vi "Terminal_Log_In_Judge.vi"(8 "密码":string, 9 "用户名":string, 10 "用户个数":dbl, 11 "用户名密码信息":string[][](table)) -> (3 "用户名密码匹配":bool)   [LabVIEW 2014]
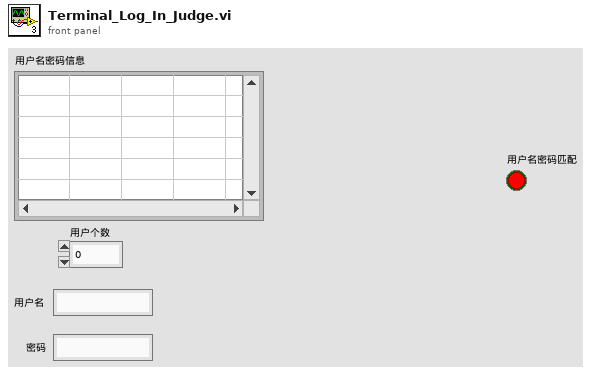
[diagram p1: front panel]
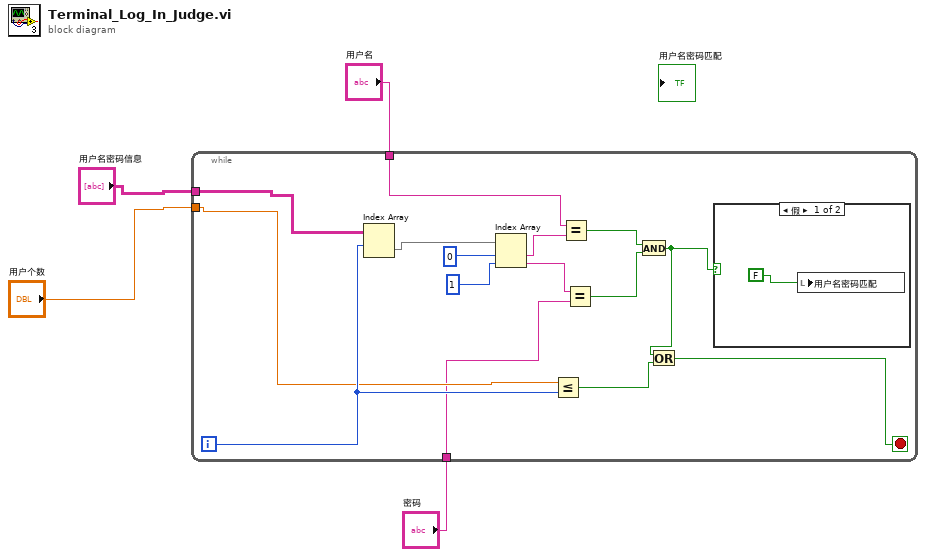
[diagram p0: block diagram]
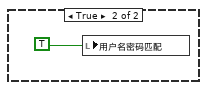
[diagram p2: hidden frame]
diagram:
  n1 = while {
    tunnel: "用户名" -> [w12]
    tunnel: "用户名密码信息" -> [w7]
    tunnel: "用户个数" -> [w6]
    tunnel: "密码" -> [w5]
    i -> [w11]
    stop <- w8 stop-if-true
    n2 = Index Array(array=w7, index (row)=w11) -> (element=w19:string[])  [unwired: 1 in]
    n3 = Index Array(array=w19, index #1=0, index #2=1) -> (element #1=w16:string, element #2=w15:string)
    n4 = Less Or Equal?(x=w6, y=w11) -> (x <= y?=w9:bool)
    n5 = Equal?(x=w12, y=w16) -> (x = y?=w14:bool)
    n6 = Equal?(x=w15, y=w5) -> (x = y?=w13:bool)
    n7 = And(x=w14, y=w13) -> (x .and. y?=w10:bool)
    n8 = Or(x=w10, y=w9) -> (x .or. y?=w8:bool)
    n9 = case shown="假" w10 {
      frame False {
        n10 = local write "用户名密码匹配"(FALSE) -> ()
      }
      frame True {
        n11 = local write "用户名密码匹配"(TRUE) -> ()
      }
    }
  }
